vi "Datum Subset.vi"(8 "limit size":i32, 9 "start":i32, 10 "len":i32, 11 "data":T1[](array[typedef])) -> (0 "count of datums out":i32, 1 "datums out":T1[](array[typedef]), 2 "count of datums 1":i32, 3 "datums 1":T1[](array[typedef]))   [LabVIEW 2020, in "NI_Bytestream.lvlib" / "Bytestream.lvclass"]
uses:
  <vilib>/Array/Bytestream/Bytestream.lvclass
  <vilib>/Array/Bytestream/Datum.ctl
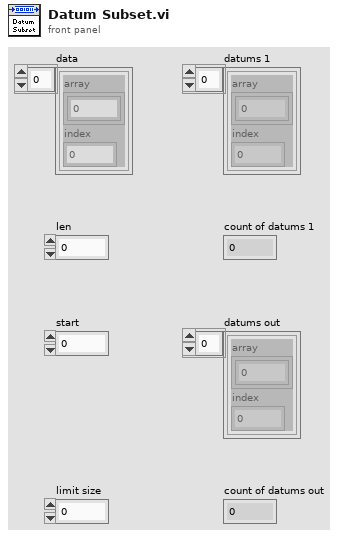
[diagram p1: front panel]
types:
  T1 = typedef "NI_Bytestream.lvlib/Bytestream.lvclass/Datum.ctl" = cluster{"array":u8[], "index":i32}
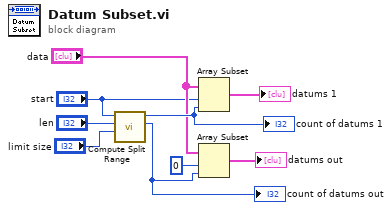
[diagram p0: block diagram]
diagram:
  n1 = call <vilib>:"Compute Split Range.vi"("limit size"="limit size", "length"="len", "start"="start") -> ("terminal length"=w7:i32, "initial length"=w8:i32)  [unwired: 7 in]
  "count of datums 1" <- w8
  "count of datums out" <- w7
  n2 = Array Subset(array="data", index="start", length=w8) -> (→"datums 1":T1[])
  n3 = Array Subset(array="data", index=0, length=w7) -> (→"datums out":T1[])
